vi "niFpga wdp fft sim main 4wire.vi"(0 "real data in":fxp<+/-,8,1>[](array[numeric])=[0.0, 0.0], 1 "reset":bool, 5 "imaginary data in":fxp<+/-,8,1>[](array[numeric])=[0.0, 0.0], 9 "input valid":bool, 12 "ready for output":bool) -> (3 "data indices":u16[](array[numeric]), 4 "real data out":fxp<+/-,29,12>[](array[numeric]), 6 "imaginary data out":fxp<+/-,29,12>[](array[numeric]), 10 "output valid":bool, 14 "ready for input":bool)   [LabVIEW 2017]
uses:
  <vilib>/rvi/Analysis/measure/FFT/config/niFpgaFFTSettings.ctl
  <vilib>/rvi/Analysis/common/niLvFpgaMspClockRate.ctl
  <vilib>/rvi/Analysis/measure/FFT/config/niFpgaFFTIOPattern.ctl
  <vilib>/rvi/Analysis/measure/FFT/config/niFpgaFFTScalingScheme.ctl
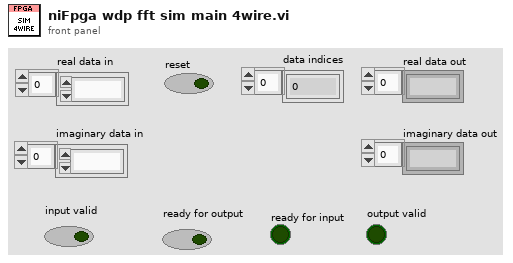
[diagram p1: front panel]
types:
  T1 = typedef "niFpgaFFTSettings.ctl" = cluster{"Number of stages":u8, "Forward?":bool, "adapt to source":bool, "Output word length":u32, "Output integer word length":i32, "Architecture":enum16{"Outside SCTL", "Inside SCTL - Burst", "Inside SCTL - Streaming"}, "input wl":u32, "input iwl":i32, "overflow?":bool, "input sign":enum32{"Signed", "Unsigned"}, "use sim models?":bool, "clock rate":T2, "pattern":T3, "mode":enum16{"Normal", "WDP"}, "scaling scheme":T4, "show enable?":bool}
  T2 = typedef "niLvFpgaMspClockRate.ctl" = enum16{"Default", "Medium", "High"}
  T3 = typedef "niFpgaFFTIOPattern.ctl" = enum16{"CI/CO", "CI/DO", "DI/CO"}
  T4 = typedef "niFpgaFFTScalingScheme.ctl" = enum16{"Unscaled", "Scaled"}
  T5 = typedef "niFpga wdp fft sim model config.ctl" = cluster{"number of stages":i32, "number of spc":i32, "Forward?":bool, "scaling scheme":T4, "internal input type":T6, "tf type":T6, "extra delay":u16, "output shift bits":i16, "reset length":u32, "input shift bits":i16, "pattern":T3}
  T6 = typedef "LVFixedPointRepBitsTypeDef.ctl" = cluster{"Signed":bool, "Word Length":u32, "Integer Word Length":i32}
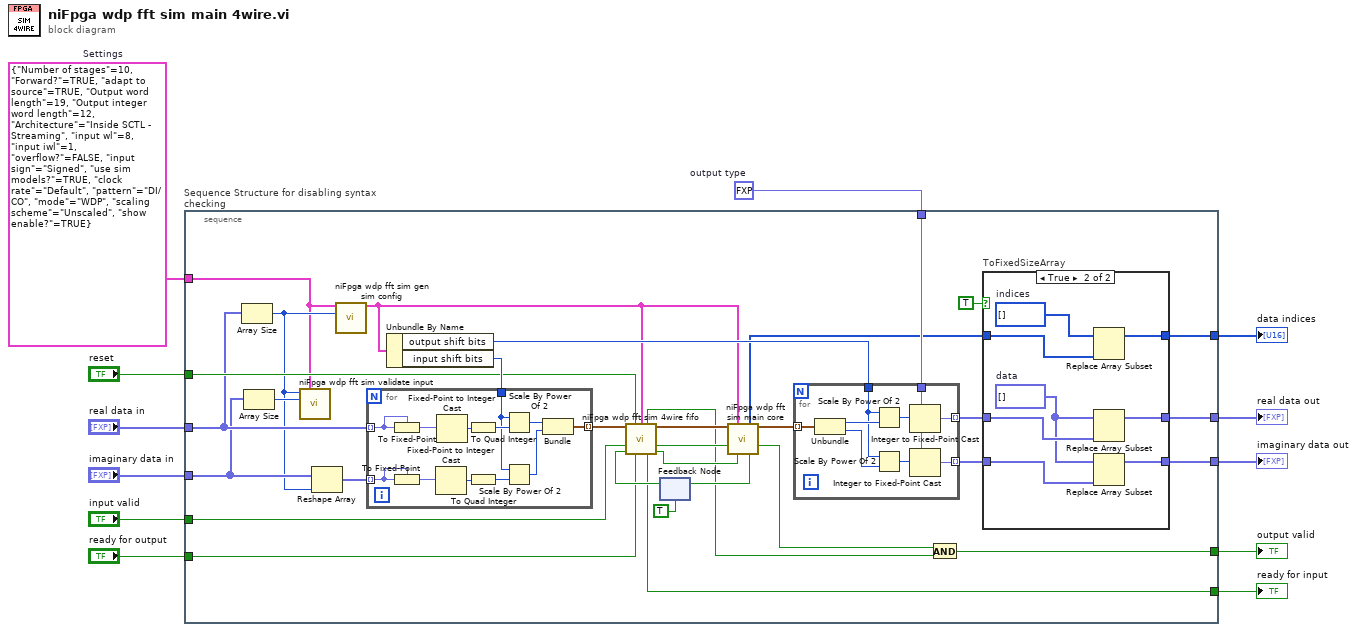
[diagram p0: block diagram]
diagram:
  w1 = fxp<+/-,19,12> 0.0  # output type
  w2 = T1 {"Number of stages"=10, "Forward?"=TRUE, "adapt to source"=TRUE, "Output word length"=19, "Output integer word length"=12, "Architecture"=enum."Inside SCTL - Streaming", "input wl"=8, "input iwl"=1, "overflow?"=FALSE, "input sign"=enum."Signed", "use sim models?"=TRUE, "clock rate"=enum."Default", "pattern"=enum."DI/CO", "mode"=enum."WDP", "scaling scheme"=enum."Unscaled", "show enable?"=TRUE}  # Settings
  n1 = stacked-sequence "Sequence Structure for disabling syntax checking" {
    tunnel: "reset" -> [w32]
    tunnel: "real data in" -> [w31]
    tunnel: "imaginary data in" -> [w25]
    tunnel: "input valid" -> [w30]
    tunnel: "ready for output" -> [w29]
    tunnel: [w28] -> w7
    tunnel: [w15] -> w6
    tunnel: [w20] -> w5
    tunnel: [w19] -> w4
    tunnel: [w17] -> w3
    tunnel: w2 -> [w13]
    tunnel: w1 -> [w27]
    frame #0 {
      n2 = Array Size(array=w31) -> (size(s)=w23:i32)
      n3 = Array Size(array=w25) -> (size(s)=w24:i32)
      n4 = call <vilib>:"niFpga wdp fft sim validate input.vi"("size of real"=w23, "FFTConfigSettings"=w13, "size of imaginary"=w24) -> ()  [unwired: 13 in]
      n5 = Reshape Array(w25, w23) -> (w26:fxp<+/-,8,1>[])
      n6 = call <vilib>:"niFpga wdp fft sim gen sim config.vi"("FFTConfigSettings"=w13, "samples/cycle"=w23) -> ("Config"=w33:T5)  [unwired: 13 in]
      n7 = Unbundle By Name(w33) -> ("output shift bits"=w36:i16, "input shift bits"=w34:i16)
      n8 = for {
        tunnel: w31 -> [w58] mode=indexing
        tunnel: w26 -> [w56] mode=indexing
        tunnel: [w65] -> w35 mode=indexing
        tunnel: w34 -> [w62]
        n9 = To Fixed-Point(fixed-point type=w58, number=w58) -> (fixed-point=w59:fxp<+/-,8,1>)
        n10 = To Fixed-Point(fixed-point type=w56, number=w56) -> (fixed-point=w57:fxp<+/-,8,1>)
        n11 = Fixed-Point to Integer Cast(1:w57) -> (0:w66:i8)
        n12 = Fixed-Point to Integer Cast(1:w59) -> (0:w67:i8)
        n13 = To Quad Integer(1:w67) -> (0:w64:i64)
        n14 = To Quad Integer(1:w66) -> (0:w63:i64)
        n15 = Scale By Power Of 2(n=w62, x=w64) -> (x*2^n=w61:i64)
        n16 = Scale By Power Of 2(n=w62, x=w63) -> (x*2^n=w60:i64)
        n17 = Bundle(w61, w60) -> (w65:cluster{i64, i64})  [unwired: 1 in]
      }
      n18 = feedback #1(TRUE ("ready for frame")) -> (w39:bool)
      n19 = call <vilib>:"niFpga wdp fft sim 4wire fifo.vi"("data in"=w35, "reset"=w32, "Config"=w33, "input valid"=w30, "ready for frame"=w39, "ready for output"=w29) -> ("not in reset"=w37:bool, "data out"=w43:cluster{"data re":i64, "data im":i64}[], "frame start"=w41:bool, "ready for input"=w28:bool, "enable"=w40:bool)  [unwired: 5 in]
      n20 = call <vilib>:"niFpga wdp fft sim main core.vi"("data in"=w43, "Config"=w33, "input frame start"=w41, "enable"=w40) -> ("data indices"=w18:u16[], "data out"=w44:cluster{"data re":i64, "data im":i64}[], "output valid"=w38:bool, "ready for frame"=w42:bool)  [unwired: 7 in, 1 out]
      n21 = feedback-in #1(w42) -> ()
      n22 = for {
        tunnel: w27 -> [w76]
        tunnel: [w75] -> w22 mode=indexing
        tunnel: [w74] -> w21 mode=indexing
        tunnel: w36 -> [w69]
        tunnel: w44 -> [w68] mode=indexing
        n23 = Unbundle(w68) -> ("data re"=w73:i64, "data im"=w70:i64)
        n24 = Scale By Power Of 2(n=w69, x=w73) -> (x*2^n=w72:i64)
        n25 = Scale By Power Of 2(n=w69, x=w70) -> (x*2^n=w71:i64)
        n26 = Integer to Fixed-Point Cast(fixed-point type=w76, integer=w72) -> (fixed-point=w75:fxp<+/-,19,12>)
        n27 = Integer to Fixed-Point Cast(fixed-point type=w76, integer=w71) -> (fixed-point=w74:fxp<+/-,19,12>)
      }
      n28 = And(x=w38, y=w37) -> (x .and. y?=w15:bool)
      n29 = case "ToFixedSizeArray" shown="True" TRUE {
        tunnel: w18 -> [w47 w55]
        tunnel: [w47 w50] -> w17
        tunnel: w22 -> [w46 w54]
        tunnel: w21 -> [w45 w53]
        tunnel: [w46 w49] -> w19
        tunnel: [w45 w48] -> w20
        frame False {
        }
        frame True {
          w51 = u16[] []  # indices
          w52 = fxp<+/-,19,2>[] []  # data
          n30 = Replace Array Subset(array=w51, new element=w55) -> (w50:u16[])  [unwired: 1 in]
          n31 = Replace Array Subset(array=w52, new element=w54) -> (w49:fxp<+/-,19,2>[])  [unwired: 1 in]
          n32 = Replace Array Subset(array=w52, new element=w53) -> (w48:fxp<+/-,19,2>[])  [unwired: 1 in]
        }
      }
    }
  }
  "ready for input" <- w7
  "output valid" <- w6
  "real data out" <- w4
  "imaginary data out" <- w5
  "data indices" <- w3
